vi "init.vi"(8 "error in (no error)":errorcluster, 11 "canon_m3 in":refnum<class "protocol_canonM3.lvclass">) -> (0 "error out":errorcluster, 3 "canon_m3 out":refnum<class "protocol_canonM3.lvclass">)   [LabVIEW 2015, in "protocol_canonM3.lvclass"]
uses:
  protocol_canonM3.lvclass
  command_click.lvclass
  command/command_generic.lvclass
  protocol_canonM3.lvclass/protocol_canonM3.ctl
  protocol_Generic/Protocol_Generic.lvclass
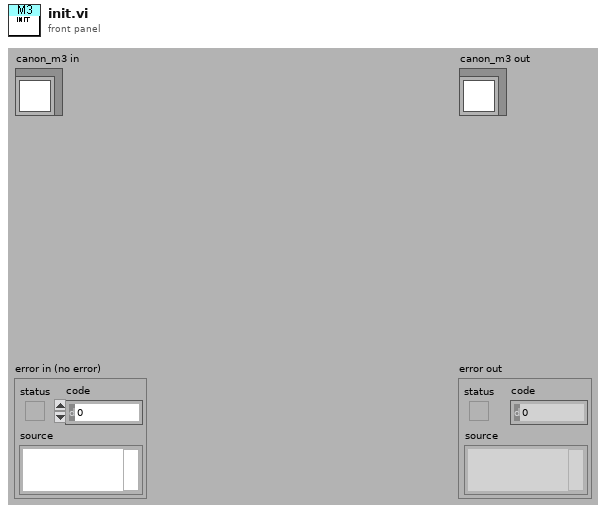
[diagram p1: front panel]
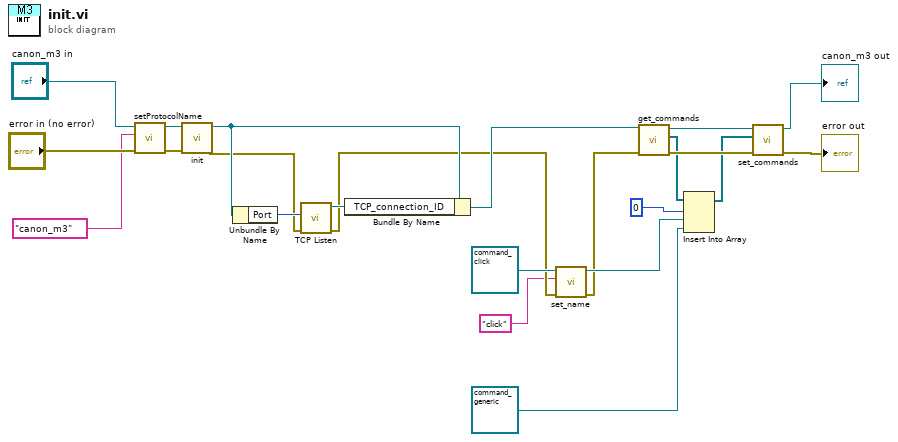
[diagram p0: block diagram]
diagram:
  n1 = call-dynamic "setProtocolName.vi"("error in (no error)"="error in (no error)", "Name"="canon_m3", "Protocol_Generic in"="canon_m3 in") -> ("error out"=w21:errorcluster, "Protocol_Generic out"=w22:refnum<class "protocol_canonM3.lvclass">)  [unwired: 7 in]
  n2 = call-parent "init.vi"("error in (no error)"=w21, "Protocol_Generic in"=w22) -> ("error out"=w7:errorcluster, "Protocol_Generic out"=w18:refnum<class "protocol_canonM3.lvclass">)  [unwired: 8 in]
  n3 = Unbundle By Name(w18) -> ("Port"=w19:i32)
  n4 = call <vilib>:"TCP Listen.vi"("error in (no error)"=w7, "port"=w19) -> ("error out"=w3:errorcluster, "connection ID"=w17:refnum<k5>)  [unwired: 5 in, 3 out]
  n5 = Bundle By Name(cluster=w18, "TCP_connection_ID"=w17) -> (w15:refnum<class "protocol_canonM3.lvclass">)
  n6 = call-dynamic "set_name.vi"("error in (no error)"=w3, "name"="click", "command in"=refnum<class "command_click.lvclass"> refnum ("command_click.lvclass")) -> ("error out"=w2:errorcluster, "command out"=w4:refnum<class "command_click.lvclass">)  [unwired: 7 in]
  n7 = call-dynamic "get_commands.vi"("error in (no error)"=w2, "Protocol_Generic in"=w15) -> ("error out"=w14:errorcluster, "commands"=w10:refnum<class "command_generic.lvclass">[], "Protocol_Generic out"=w13:refnum<class "protocol_canonM3.lvclass">)  [unwired: 7 in]
  n8 = Insert Into Array(array=w10, index=0, new element #1=w4, new element #2=refnum<class "command_generic.lvclass"> refnum ("command_generic.lvclass")) -> (w8:refnum<class "command_generic.lvclass">[])
  n9 = call-dynamic "set_commands.vi"("error in (no error)"=w14, "commands"=w8, "Protocol_Generic in"=w13) -> ("error out"=→"error out":errorcluster, "Protocol_Generic out"=→"canon_m3 out":refnum<class "protocol_canonM3.lvclass">)  [unwired: 7 in]
